vi "Destroy Reference.vi"(8 "Error In":errorcluster, 11 "Writer In":refnum<data-value>) -> (0 "Error Out":errorcluster, 3 "Writer Out":refnum<class "Writer.lvclass">)   [LabVIEW 2018, in "Toolkit.lvlib" / "Writer.lvclass"]
doc: "Destroys a reference to a Writer class object. This may free resources associated with the reference but not necessarily the object."
uses:
  Writer.lvclass
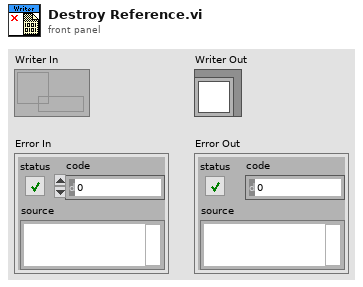
[diagram p1: front panel]
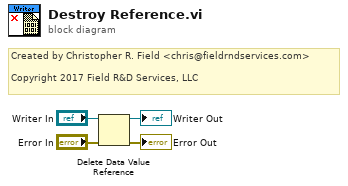
[diagram p0: block diagram]
diagram:
  # "Created by Christopher R. Field <chris@fieldrndservices.com>\n\nCopyright 2017 Field R&D Services, LLC"
  n1 = Delete Data Value Reference(data value reference="Writer In", error in="Error In") -> (data value=→"Writer Out":refnum<class "Writer.lvclass">, error out=→"Error Out":errorcluster)
